vi "Controller - SEND - Message.vi"(7 "Destination":T1, 8 "error in":errorcluster) -> (0 "error out":errorcluster)   [LabVIEW 2023, in "Controller.lvlib" / "Controller.lvclass"]
uses:
  Controller.lvclass
  Controller - Ctrl - Actor - Destination.ctl
  Message_Distributor/Message_Distributor_Class.lvclass
  Users/rodrigoarguelloserrano/UofA_Bootcamp/Challanges/LV_AF_Project/AF_Architecture/Abstraction_Interface_Class/Abstraction_Interface_Class.lvclass
  GUI/GUI_Class.lvclass
  Console/Console_Class.lvclass
  Controller - Ctrl - FGV - Action.ctl
  SW_Interface/SW_Interface_Class.lvclass
  Message_Distributor/Distributor_Class Messages/Distributor - SEND - Triggered Event Msg/Distributor - SEND - Triggered Event Msg.lvclass/Distributor - SEND - Triggered Event Msg.ctl
  <vilib>/ActorFramework/Message Enqueuer/Message Enqueuer.lvclass/Message Enqueuer.ctl
  <vilib>/ActorFramework/Message Enqueuer/Enqueue.vi
  Message_Distributor/Distributor_Class Messages/Distributor - SEND - Triggered Event Msg/Distributor - SEND - Triggered Event Msg.lvclass
  Applications/National Instruments/LabVIEW 2023 64-bit/vi.lib/ActorFramework/Message/Message.lvclass
  <vilib>/ActorFramework/Message Priority Queue/Priority Enqueue.vi
  Abstraction_Interface_Class/Abstraction_Interface_Class.lvclass
panel:
  in  "Value":string
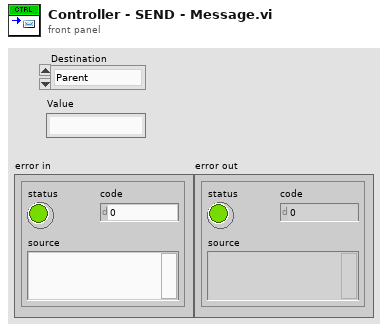
[diagram p1: front panel]
types:
  T1 = typedef "Controller.lvlib/Controller.lvclass/Controller - Ctrl - Actor - Destination.ctl" = enum16{"Parent", "Child_1", "Child_2", "Child_3"}
  T2 = typedef "Controller.lvlib/Controller.lvclass/Controller - Ctrl - FGV - Action.ctl" = enum16{"Int", "Get"}
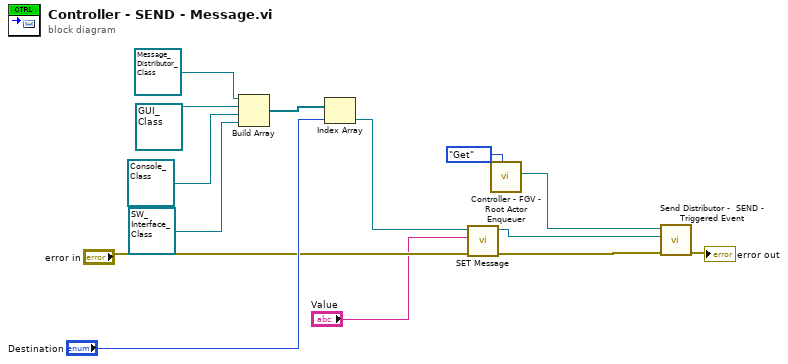
[diagram p0: block diagram]
diagram:
  n1 = Build Array(refnum<class "Message_Distributor_Class.lvclass"> refnum ("Actor_Parent.lvlib:Parent_Class.lvclass"), refnum<class "GUI_Class.lvclass"> refnum ("Actor_Child_1.lvlib:Child_1_Class.lvclass"), refnum<class "Console_Class.lvclass"> refnum ("Actor_Child_2.lvlib:Child_2_Class.lvclass"), refnum<class "SW_Interface_Class.lvclass"> refnum ("Actor_Child_3.lvlib:Child_3_Class.lvclass")) -> (w11:refnum<class "Abstraction_Interface_Class.lvclass">[])
  n2 = Index Array(array=w11, index="Destination") -> (element=w1:refnum<class "Abstraction_Interface_Class.lvclass">)
  n3 = call-dynamic "SET Message.vi"("error in (no error)"="error in", "Data"="Value", "Interface_Class in"=w1) -> ("error out"=w7:errorcluster, "Interface_Class out"=w6:refnum<class "Abstraction_Interface_Class.lvclass">)  [unwired: 7 in]
  n4 = call "Controller - FGV - Root Actor Enqueuer.vi"("Action"=Controller_-_Ctrl_-_FGV_-_Action."Get") -> ("Root Enqueuer"=w4:refnum<class "Message Enqueuer.lvclass">)  [unwired: 9 in, 1 out]
  n5 = call "Send Distributor -  SEND - Triggered Event.vi"("error in (no error)"=w7, "Actor_Interface.lvlib:Interface_Class.lvclass"=w6, "Message Enqueuer"=w4) -> ("error out"=→"error out":errorcluster)  [unwired: 7 in, 1 out]
